vi "SendCommands.vi"(8 "error in (no error)":errorcluster, 11 "DAQList in":refnum<class "DAQList.lvclass">) -> (0 "error out":errorcluster, 2 "CAN Frames":T1[](array[typedef]) {"payload" format="%x"; "timestamp" format="%<%.7X\n%x>T"; "type" items=["CAN Data"=0, "CAN Remote"=1, "CAN Bus Error"=2, "CAN 2.0 Data"=8, "CAN FD Data"=16, "CAN FD+BRS Data"=24, "J1939 Data"=192, "Delay"=224, "Log Trigger"=225, "Start Trigger"=226]; "identifier" format="%x"}, 3 "DAQList out":refnum<class "DAQList.lvclass">)   [LabVIEW 2019, in "XCP_DaqDtoId.lvlib" / "DAQList.lvclass"]
uses:
  DAQList.lvclass
  <vilib>/xnet/xnet.llb/XNET Frame CAN.ctl
  <vilib>/xnet/xnet.llb/XNET Frame Type CAN.ctl
  DAQList.lvclass/DAQList.ctl
  <vilib>/ECUMC/ECUMC.llb/MC StartStop Mode.ctt
  <vilib>/ECUMC/ECUMC.llb/MC DAQ Mode.ctt
  <vilib>/xnet/xnet.llb/XNET Create Session (Frame Input Stream).vi
  <vilib>/xnet/xnet.llb/XNET Read (Frame CAN).vi
  <vilib>/ECUMC/ECUMC.lvlib
  <resource>/objmgr/xnet.rc
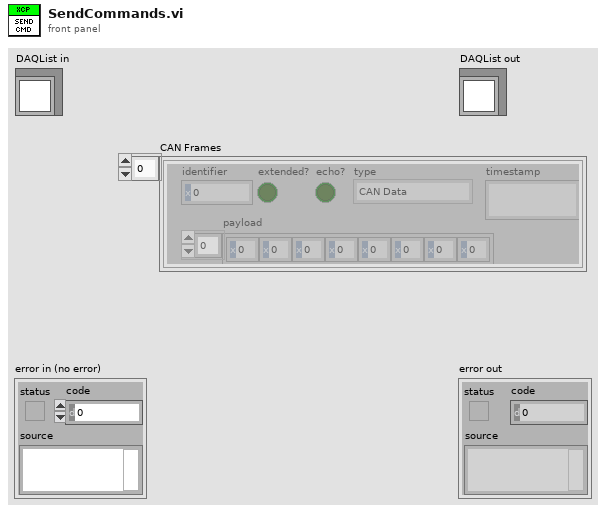
[diagram p1: front panel]
types:
  T1 = typedef "XNET Frame CAN.ctl" = cluster{"timestamp":timestamp, "payload":u8[], "identifier":u32, "type":T2, "extended?":bool, "echo?":bool}
  T2 = typedef "XNET Frame Type CAN.ctl" = u8
  T3 = typedef "ECUMC.lvlib/MC StartStop Mode.ctt" = i32
  T4 = typedef "ECUMC.lvlib/MC DAQ Mode.ctt" = i32
  T5 = typedef "ECUMC.lvlib/MC Reference.ctt" = u32
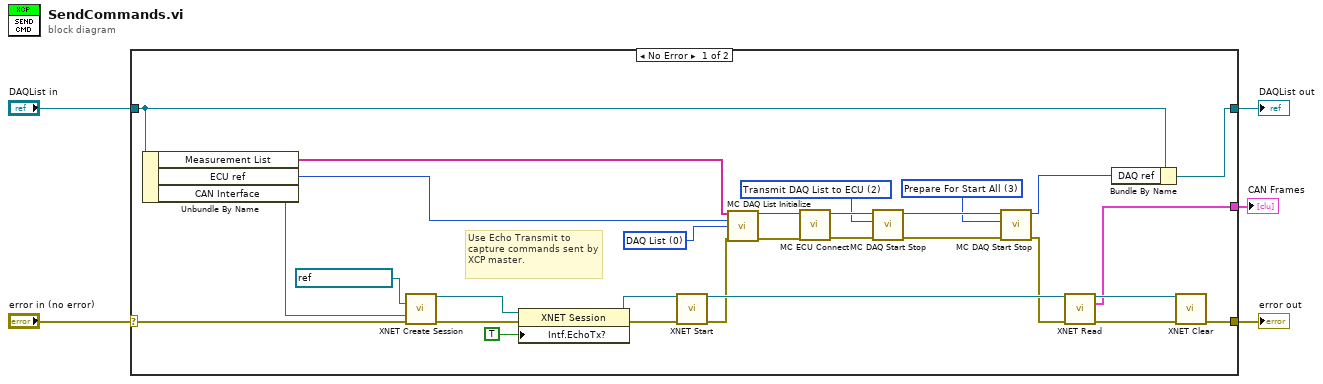
[diagram p0: block diagram]
diagram:
  n1 = case shown="No Error" "error in (no error)" {
    selector: "error in (no error)" -> [w8 w36]
    tunnel: [w7 w36] -> w4
    tunnel: [w13 w35] -> w2
    tunnel: "DAQList in" -> [w14 w35]
    tunnel: [w6 _] -> w1
    frame No Error {
      w15 = T3 3 items=["Stop DAQ List", "Start DAQ List", "Transmit DAQ List to ECU", "Prepare For Start All", "Start All DAQ Lists", "Stop All DAQ Lists"] ("mode")
      w23 = T3 2 items=["Stop DAQ List", "Start DAQ List", "Transmit DAQ List to ECU", "Prepare For Start All", "Start All DAQ Lists", "Stop All DAQ Lists"] ("mode")
      w22 = T4 0 items=["DAQ List", "Polling", "STIM List", "time stamped read"] ("mode")
      # "Use Echo Transmit to capture commands sent by XCP master."
      n2 = Unbundle By Name(w14) -> ("Measurement List"=w11:string[], "ECU ref"=w10:T5, "CAN Interface"=w9:refnum<k21>)
      n3 = call-poly <vilib>:"XNET Create Session.vi"("cluster (:memory:)"=refnum<k21> ":subordinate:", "interface"=w9, "error in (no error)"=w8) -> ("session out"=w31:refnum<k21>, "error out"=w30:errorcluster)  [unwired: 11 out]
      n4 = property class="XNET Session"(reference=w31, error in=w30, "Intf.EchoTx?"=TRUE ("Interface:Echo Transmit?")) -> (reference out=w32:refnum<k21>, error out=w33:errorcluster)
      n5 = call <vilib>:"XNET Start.vi"("session in"=w32, "error in (no error)"=w33) -> ("session out"=w25:refnum<k21>, "error out"=w24:errorcluster)  [unwired: 12 in]
      n6 = call <vilib>:"MC DAQ List Initialize.vi"("measurement list"=w11, "ECU ref in"=w10, "mode"=w22, "error in"=w24) -> ("DAQ ref out"=w21:T5, "error out"=w27:errorcluster)  [unwired: 10 in]
      n7 = call <vilib>:"MC ECU Connect.vi"("error in"=w27, "ECU ref in"=w21) -> ("error out"=w28:errorcluster, "ECU ref out"=w26:T5)  [unwired: 8 in]
      n8 = call <vilib>:"MC DAQ Start Stop.vi"("error in"=w28, "mode"=w23, "DAQ ref in"=w26) -> ("error out"=w17:errorcluster, "DAQ ref out"=w18:T5)  [unwired: 7 in]
      n9 = call <vilib>:"MC DAQ Start Stop.vi"("error in"=w17, "mode"=w15, "DAQ ref in"=w18) -> ("error out"=w16:errorcluster, "DAQ ref out"=w12:T5)  [unwired: 7 in]
      n10 = call-poly <vilib>:"XNET Read.vi"("session in"=w25, "error in (no error)"=w16) -> ("session out"=w20:refnum<k21>, "data"=w6:T1[], "error out"=w19:errorcluster)  [unwired: 11 out]
      n11 = Bundle By Name(cluster=w14, "DAQ ref"=w12) -> (w13:refnum<class "DAQList.lvclass">)
      n12 = call <vilib>:"XNET Clear.vi"("session in"=w20, "error in (no error)"=w19) -> ("error out"=w7:errorcluster)  [unwired: 13 in]
    }
    frame Error {
    }
  }
  "error out" <- w4
  "DAQList out" <- w2
  "CAN Frames" <- w1
